vi "ADC Command.vi"(0 "object in":refnum<class "Serial Device.lvclass">, 1 "Marca":string, 5 "Canal":string(combo), 11 "error in (no error)":errorcluster) -> (4 "object out":refnum<class "Serial Device.lvclass">, 6 "Command":string, 10 "Expected response":string, 15 "error out":errorcluster)   [LabVIEW 2020, in "Serial Device.lvclass"]
uses:
  Serial Device.lvclass
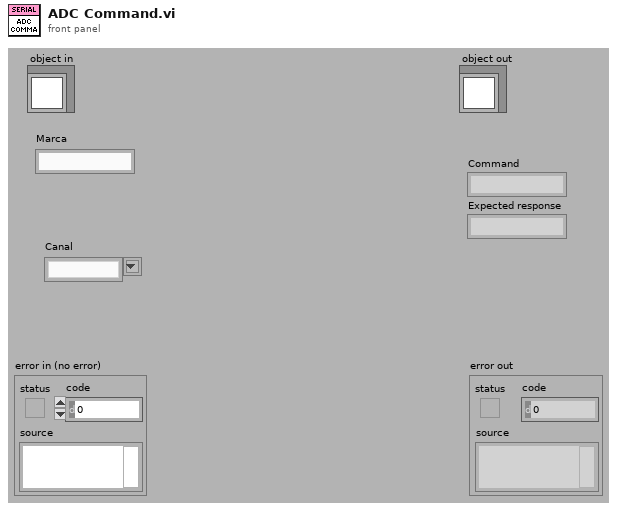
[diagram p1: front panel]
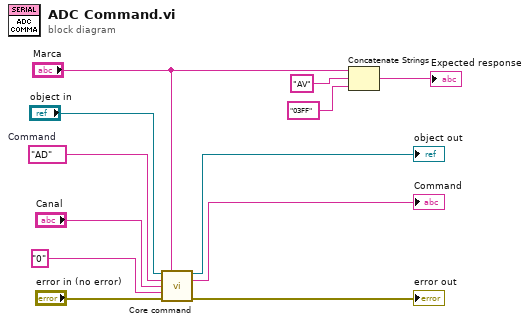
[diagram p0: block diagram]
diagram:
  w11 = "AD"  # Command
  n1 = call-dynamic "Core command.vi"("object in"="object in", "Marca"="Marca", "Command"=w11, "Param 1"="Canal", "Param 2"="0", "error in (no error)"="error in (no error)") -> ("object out"=→"object out":refnum<class "Serial Device.lvclass">, "Command"=→"Command":string, "error out"=→"error out":errorcluster)  [unwired: 6 in, 1 out]
  n2 = Concatenate Strings("Marca", "AV" ("string"), "03FF" ("string")) -> (→"Expected response":string)
